vi "ClearPortList.vi"(1 "topic port":u16, 2 "ROS":T1={"topic port"=0, "Node"="", "topic"="", "type"="", "node port"=0, "error "={"status"=FALSE, "code"=0, "source"=""}, "Direction"=enum."Node", "Update (ms)"=1, "FIFO size"=1}) -> ()   [LabVIEW 2015]
doc: "Clears a port from the server port list"
uses:
  _ROSControl.ctl
  _ROSDirection.ctl
  _ROSDefinition.vi
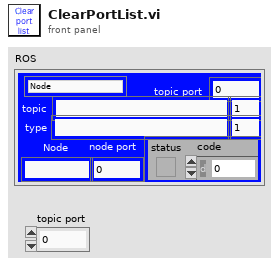
[diagram p1: front panel]
types:
  T1 = typedef "_ROSControl.ctl" = cluster{"topic port":u16, "Node":string, "topic":string, "type":string, "node port":u16, "error ":errorcluster, "Direction":T2, "Update (ms)":u16, "FIFO size":u16}
  T2 = typedef "_ROSDirection.ctl" = enum16{"Node", "Publisher", "Subscriber", "ServiceClient", "ServiceProvider"}
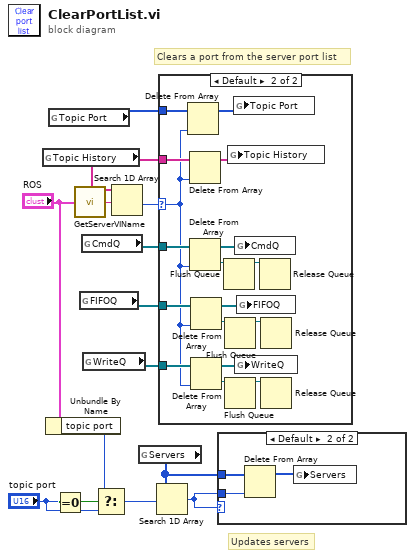
[diagram p0: block diagram]
diagram:
  # "Updates servers"
  # "Clears a port from the server port list"
  n1 = global read "_ROSDefinition.vi" "Topic History"() -> (w11:string[])
  n2 = Unbundle By Name("ROS") -> ("topic port"=w6:u16)
  n3 = global read "_ROSDefinition.vi" "Topic Port"() -> (w10:u16[])
  n4 = Equal To 0?(x="topic port") -> (x = 0?=w8:bool)
  n5 = call "GetServerVIName.vi"("ROS"="ROS") -> ("vi name"=w9:string)
  n6 = global read "_ROSDefinition.vi" "FIFOQ"() -> (w2:refnum<queue>[])
  n7 = global read "_ROSDefinition.vi" "CmdQ"() -> (w3:refnum<queue>[])
  n8 = global read "_ROSDefinition.vi" "WriteQ"() -> (w1:refnum<queue>[])
  n9 = Select(t=w6, s=w8, f="topic port") -> (s? t:f=w4:u16)
  n10 = Search 1D Array(1D array=w11, element=w9) -> (index of element=w12:i32)  [unwired: 1 in]
  n11 = global read "_ROSDefinition.vi" "Servers"() -> (w14:u16[])
  n12 = Search 1D Array(1D array=w14, element=w4) -> (index of element=w13:i32)  [unwired: 1 in]
  n13 = case shown="Default" w12 {
    selector: w12 -> [_ w15]
    tunnel: w11 -> [_ w31]
    tunnel: w10 -> [_ w28]
    tunnel: w3 -> [_ w27]
    tunnel: w2 -> [_ w22]
    tunnel: w1 -> [_ w16]
    frame -1 {
    }
    frame Default {
      n14 = Delete From Array(array=w28, index=w15) -> (array with subset deleted=w29:u16[])  [unwired: 1 in, 1 out]
      n15 = Delete From Array(array=w31, index=w15) -> (array with subset deleted=w30:string[])  [unwired: 1 in, 1 out]
      n16 = Delete From Array(array=w27, index=w15) -> (deleted portion=w25:refnum<queue>, array with subset deleted=w26:refnum<queue>[])  [unwired: 1 in]
      n17 = Delete From Array(array=w22, index=w15) -> (deleted portion=w24:refnum<queue>, array with subset deleted=w23:refnum<queue>[])  [unwired: 1 in]
      n18 = Delete From Array(array=w16, index=w15) -> (deleted portion=w17:refnum<queue>, array with subset deleted=w18:refnum<queue>[])  [unwired: 1 in]
      n19 = Flush Queue(queue=w25) -> (queue out=w21:refnum<queue>)  [unwired: 1 in, 2 out]
      n20 = Flush Queue(queue=w24) -> (queue out=w20:refnum<queue>)  [unwired: 1 in, 2 out]
      n21 = Flush Queue(queue=w17) -> (queue out=w19:refnum<queue>)  [unwired: 1 in, 2 out]
      n22 = global write "_ROSDefinition.vi" "Topic History"(w30) -> ()
      n23 = global write "_ROSDefinition.vi" "Topic Port"(w29) -> ()
      n24 = global write "_ROSDefinition.vi" "CmdQ"(w26) -> ()
      n25 = global write "_ROSDefinition.vi" "WriteQ"(w18) -> ()
      n26 = global write "_ROSDefinition.vi" "FIFOQ"(w23) -> ()
      n27 = Release Queue(queue=w21) -> ()  [unwired: 2 in, 3 out]
      n28 = Release Queue(queue=w20) -> ()  [unwired: 2 in, 3 out]
      n29 = Release Queue(queue=w19) -> ()  [unwired: 2 in, 3 out]
    }
  }
  n30 = case shown="Default" w13 {
    tunnel: w13 -> [_ w32]
    tunnel: w14 -> [_ w34]
    frame -1 {
    }
    frame Default {
      n31 = Delete From Array(array=w34, index=w32) -> (array with subset deleted=w33:u16[])  [unwired: 1 in, 1 out]
      n32 = global write "_ROSDefinition.vi" "Servers"(w33) -> ()
    }
  }
